vi "Simple Reader.vi"(8 "error in (no error)":errorcluster, 11 "Stepper in":refnum<class "Stepper.lvclass">) -> (0 "error out":errorcluster, 2 "Signals":dbl[](array[numeric]), 3 "Stepper out":refnum<class "Stepper.lvclass">)   [LabVIEW 2018, in "Stepper.lvclass"]
uses:
  Stepper.lvclass
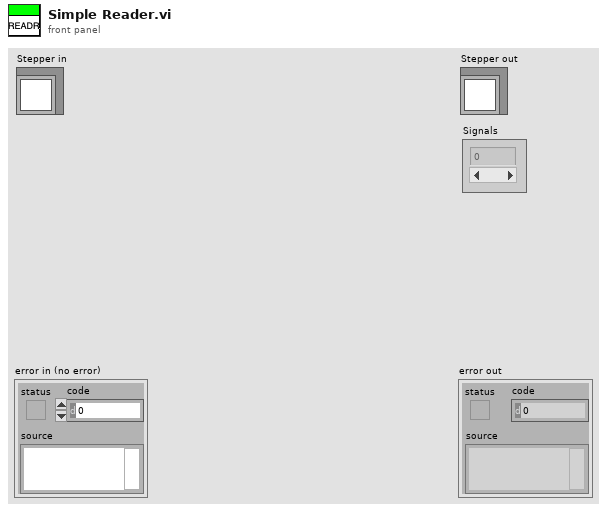
[diagram p1: front panel]
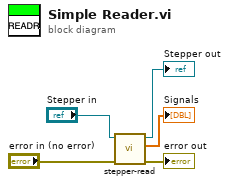
[diagram p0: block diagram]
diagram:
  n1 = call "stepper-read.vi"("error in (no error)"="error in (no error)", "Stepper.lvclass"="Stepper in") -> ("error out"=→"error out":errorcluster, "Result"=→"Signals":dbl[], "Stepper.lvclass Out"=→"Stepper out":refnum<class "Stepper.lvclass">)  [unwired: 7 in]
